vi "Delay.vi"(7 "milliseconds to wait":u32, 8 "error in (no error)":errorcluster, 11 "VISA Refnum  In":refnum<visa-resource-name>) -> (0 "error out":errorcluster, 3 "VISA Refnum out":refnum<visa-resource-name>)   [LabVIEW 2020]
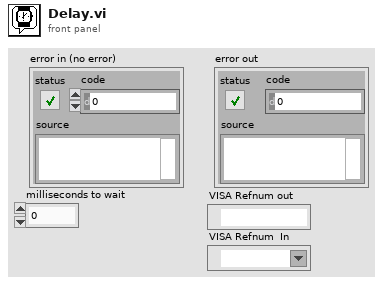
[diagram p1: front panel]
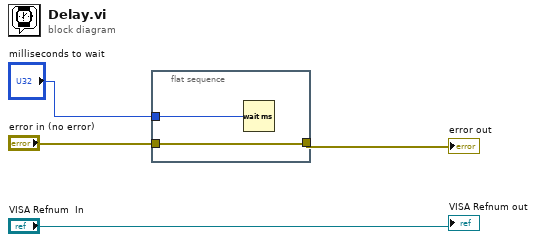
[diagram p0: block diagram]
diagram:
  n1 = flat-sequence {
    tunnel: [w6] -> w4
    tunnel: "error in (no error)" -> [w6]
    tunnel: "milliseconds to wait" -> [w5]
    frame #0 {
      n2 = Wait (ms)(milliseconds to wait=w5) -> ()  [unwired: 1 out]
    }
  }
  "error out" <- w4
  "VISA Refnum out" <- "VISA Refnum  In"
